vi "HEWH Serial Data Read.vi"(0 "Serial Port Ref":refnum<visa-resource-name>="COM3", 2 "GEA2 HyperData":bool, 5 "Retries":i32=1, 7 "Serial Port Available?":bool=TRUE, 11 "error in (no error)":errorcluster, 13 "Enable Clear Buf.":bool=TRUE) -> (4 "Serial Read OK":bool, 6 "Read String":string, 8 "Retries":i32, 15 "error out":errorcluster)   [LabVIEW 2012]
uses:
  Global HEWH.vi
panel:
  in  "Maxretry":u32
  in  "Maxtime":u32
  out "Time":u32
  out "Serial Settings:Number of Bytes at Serial Port":u32
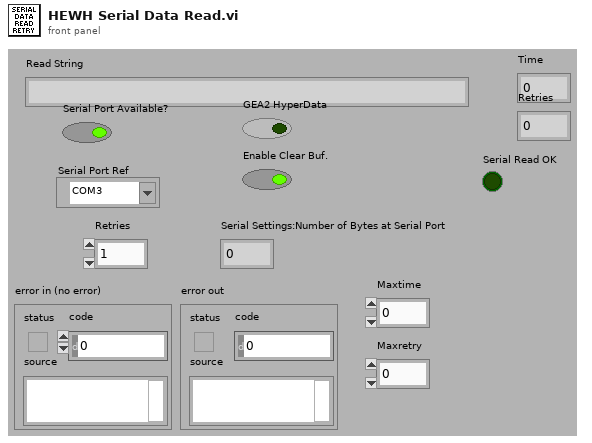
[diagram p1: front panel]
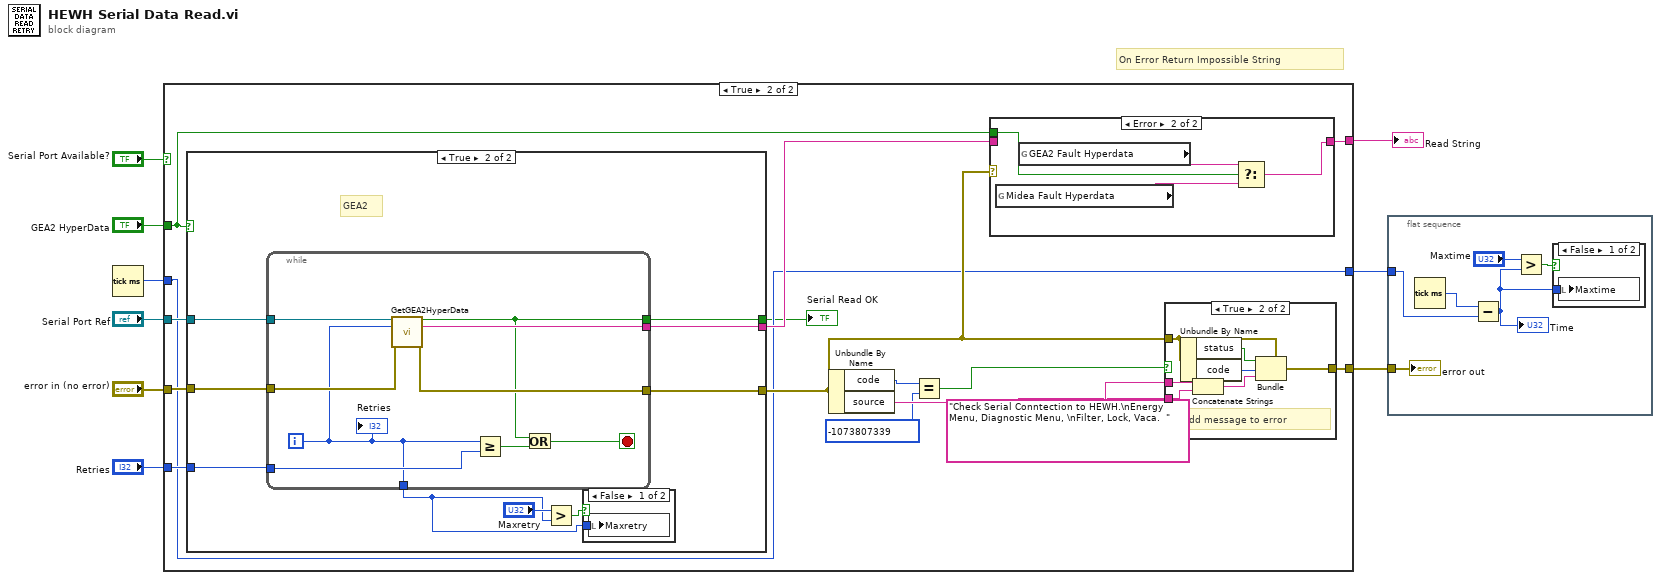
[diagram p0: block diagram]
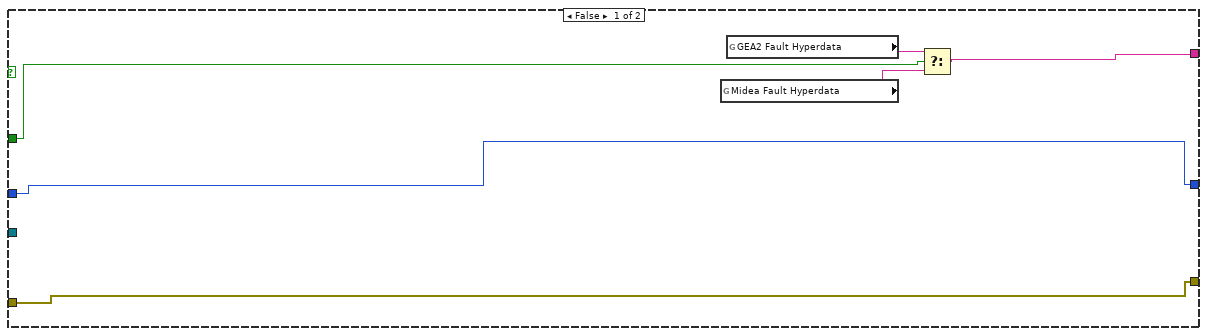
[diagram p3: hidden frame]
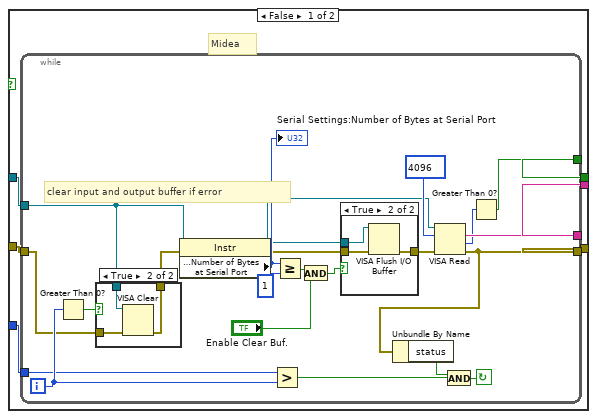
[diagram p4: hidden frame]
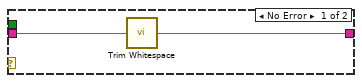
[diagram p8: hidden frame]
diagram:
  # "On Error Return Impossible String"
  n1 = Tick Count (ms)() -> (millisecond timer value=w2:u32)
  n2 = case shown="True" "Serial Port Available?" {
    tunnel: [w10 w26] -> w9
    tunnel: "Serial Port Ref" -> [_ w23]
    tunnel: "error in (no error)" -> [w15 w22]
    tunnel: [w15 w20] -> w5
    tunnel: "Retries" -> [_ w19]
    tunnel: "GEA2 HyperData" -> [w11 w16]
    tunnel: w2 -> [w14 w18]
    tunnel: [w14 w18] -> w1
    frame False {
      n3 = global read "Global HEWH.vi" "Midea Fault Hyperdata"() -> (w13:string)
      n4 = global read "Global HEWH.vi" "GEA2 Fault Hyperdata"() -> (w12:string)
      n5 = Select(t=w12, s=w11, f=w13) -> (s? t:f=w10:string)
    }
    frame True {
      n6 = case shown="True" w16 {
        tunnel: [w36 w72] -> w30
        tunnel: w23 -> [w35 w75]
        tunnel: w22 -> [w34 w74]
        tunnel: [w33 w71] -> w21
        tunnel: w19 -> [w32 w73]
        tunnel: [w31 w70] -> w17
        frame False {
          # "Midea"
          n7 = while {
            tunnel: [w57] -> w36
            tunnel: [w51] -> w33
            tunnel: w35 -> [w43]
            tunnel: w34 -> [w45]
            tunnel: w32 -> [w42]
            tunnel: [w37] -> w31
            i -> [w47]
            stop <- w48 continue-if-true
            # "clear input and output buffer if error"
            n8 = Greater Than 0?(x=w47) -> (x > 0?=w46:bool)
            n9 = case shown="True" w46 {
              tunnel: w43 -> [_ w62]
              tunnel: w45 -> [w59 w61]
              tunnel: [w59 w60] -> w44
              frame False {
              }
              frame True {
                n10 = VISA Clear(VISA resource name=w62, error in (no error)=w61) -> (error out=w60:errorcluster)  [unwired: 1 out]
              }
            }
            n11 = property class="Instr"(reference=w43, error in=w44) -> (reference out=w54:refnum<visa-resource-name>, error out=w53:errorcluster, "Serial Settings:Number of Bytes at Serial Port"=w56:u32)
            "Serial Settings:Number of Bytes at Serial Port" <- w56
            n12 = Greater?(x=w42, y=w47) -> (0:w49:bool)
            n13 = Greater Or Equal?(x=w56, y=u32 1) -> (x >= y?=w41:bool)
            n14 = And(x=w41, y="Enable Clear Buf.") -> (x .and. y?=w40:bool)
            n15 = case shown="True" w40 {
              tunnel: w54 -> [_ w66]
              tunnel: w53 -> [w63 w65]
              tunnel: [w63 w64] -> w52
              frame False {
              }
              frame True {
                n16 = VISA Flush I/O Buffer(VISA resource name=w66, error in (no error)=w65) -> (error out=w64:errorcluster)  [unwired: 1 in, 1 out]
              }
            }
            n17 = VISA Read(VISA resource name=w54, byte count=u32 4096, error in (no error)=w52) -> (read buffer=w57:string, return count=w38:u32, error out=w51:errorcluster)  [unwired: 1 out]
            n18 = Unbundle By Name(w51) -> ("status"=w50:bool)
            n19 = And(x=w50, y=w49) -> (x .and. y?=w48:bool)
            n20 = Greater Than 0?(x=w38) -> (x > 0?=w37:bool)
          }
        }
        frame True {
          # "GEA2"
          n21 = while {
            tunnel: w75 -> [w85]
            tunnel: w74 -> [w84]
            tunnel: w73 -> [w83]
            tunnel: [w81] -> w72
            tunnel: [w80] -> w71
            tunnel: [w78] -> w70
            tunnel: [w77] -> w67
            i -> [w77]
            stop <- w79 stop-if-true
            n22 = call "GetGEA2HyperData.vi"("ComPort"=w85, "Retry"=w77, "Error In"=w84) -> ("CRC"=w78:bool, "GEA2 Hyperdata"=w81:string, "Error Out"=w80:errorcluster)  [unwired: 10 in]
            n23 = Greater Or Equal?(x=w77, y=w83) -> (x >= y?=w82:bool)
            n24 = Or(x=w78, y=w82) -> (x .or. y?=w79:bool)
            "Retries" <- w77
          }
          n25 = Greater?(x="Maxretry", y=w67) -> (0:w68:bool)
          n26 = case shown="False" w68 {
            tunnel: w67 -> [w76 _]
            frame False {
              n27 = local write "Maxretry"(w76) -> ()
            }
            frame True {
            }
          }
        }
      }
      "Serial Read OK" <- w17
      n28 = Unbundle By Name(w21) -> ("code"=w29:i32, "source"=w25:string)
      n29 = Equal?(x=w29, y=-1073807339 ("code")) -> (x = y?=w27:bool)
      n30 = case shown="Error" w21 {
        tunnel: w30 -> [w87 _]
        tunnel: [w86 w90] -> w26
        tunnel: w16 -> [_ w91]
        frame No Error {
          n31 = call <vilib>:"Trim Whitespace.vi"("string"=w87) -> ("trimmed string"=w86:string)  [unwired: 1 in]
        }
        frame Error {
          n32 = global read "Global HEWH.vi" "Midea Fault Hyperdata"() -> (w88:string)
          n33 = global read "Global HEWH.vi" "GEA2 Fault Hyperdata"() -> (w89:string)
          n34 = Select(t=w89, s=w91, f=w88) -> (s? t:f=w90:string)
        }
      }
      n35 = case shown="True" w27 {
        tunnel: "Check Serial Conntection to HEWH.\nEnergy Menu, Diagnostic Menu, \nFilter, Lock, Vaca.  " ("error source (\" \")") -> [_ w98]
        tunnel: w25 -> [_ w99]
        tunnel: w21 -> [w92 w95]
        tunnel: [w92 w96] -> w20
        frame False {
        }
        frame True {
          # "Add message to error"
          n36 = Unbundle By Name(w95) -> ("status"=w97:bool, "code"=w93:i32)
          n37 = Concatenate Strings(w98, w99) -> (w94:string)
          n38 = Bundle(cluster=w95, "status"=w97, "code"=w93, "source"=w94) -> (w96:errorcluster)
        }
      }
    }
  }
  "Read String" <- w9
  n39 = flat-sequence {
    tunnel: w5 -> [w103]
    tunnel: w1 -> [w104]
    frame #0 {
      n40 = Tick Count (ms)() -> (millisecond timer value=w105:u32)
      n41 = Subtract(x=w105, y=w104) -> (x-y=w100:u32)
      "Time" <- w100
      n42 = Greater?(x="Maxtime", y=w100) -> (0:w101:bool)
      n43 = case shown="False" w101 {
        tunnel: w100 -> [w106 _]
        frame False {
          n44 = local write "Maxtime"(w106) -> ()
        }
        frame True {
        }
      }
      "error out" <- w103
    }
  }
